vi "construct.vi"(8 "error in (no error)":errorcluster, 9 "configuration name":string, 10 "load config file?":bool=TRUE, 11 "GenericPlugin in":refnum<class "ScanHeadMH100729FPGA.lvclass">) -> (0 "error out":errorcluster, 3 "GenericPlugin out":refnum<class "ScanHeadMH100729FPGA.lvclass">)   [LabVIEW 2010, in "ScanHeadMH100729FPGA.lvclass"]
uses:
  ScanHeadMH100729FPGA.lvclass
  GenericScanHead/GenericScanHead/GenericScanHead.lvclass
  ScanHeadMH100729FPGA.lvclass/ScanHeadMH100729FPGA.ctl
  common/classes/ErrorController/ErrorController/class_data.vi
  common/classes/GenericComponent/GenericComponent/GenericComponent.lvclass
  common/classes/ErrorController/ErrorController/ErrorController.lvclass
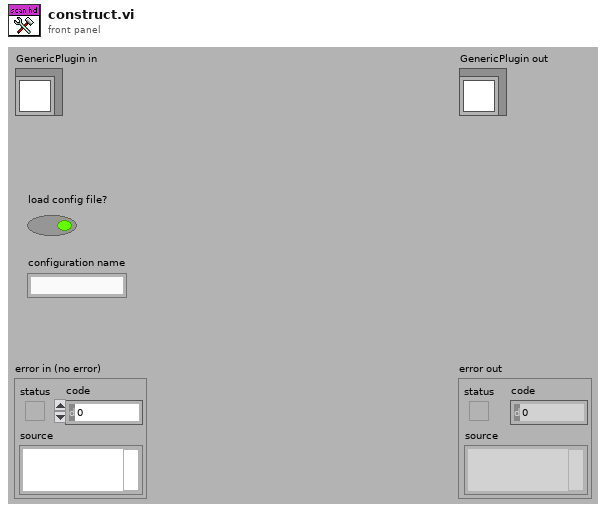
[diagram p1: front panel]
types:
  T1 = typedef "plugin_specification.ctl" = cluster{"class path":string, "configuration":string, "label":string, "settings name":string}
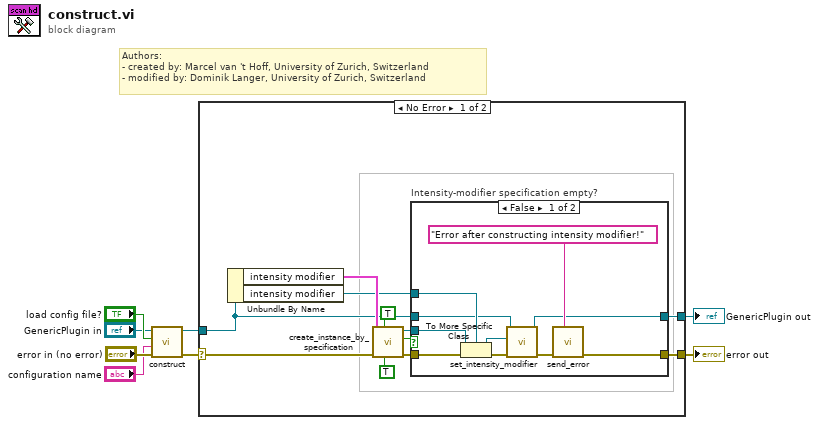
[diagram p0: block diagram]
diagram:
  # "Authors: \n- created by: Marcel van 't Hoff, University of Zurich, Switzerland\n- modified by: Dominik Langer, University of Zurich, Switzerland"
  n1 = call-parent "construct.vi"("error in (no error)"="error in (no error)", "configuration name"="configuration name", "load config file?"="load config file?", "GenericPlugin in"="GenericPlugin in") -> ("error out"=w4:errorcluster, "GenericPlugin out"=w1:refnum<class "ScanHeadMH100729FPGA.lvclass">)  [unwired: 6 in]
  n2 = case shown="No Error" w4 {
    selector: w4 -> [w12 w33]
    tunnel: [w15 w33] -> w3
    tunnel: [w9 w32] -> w2
    tunnel: w1 -> [w10 w32]
    frame No Error {
      n3 = Unbundle By Name(w10) -> ("intensity modifier"=w19:T1, "intensity modifier"=w11:refnum<class "GenericAnalogOut.lvclass">)
      n4 = call "create_instance_by_specification.vi"("be tolerant against empty specification?"=TRUE, "call constructor?"=TRUE, "error in (no error)"=w12, "component specification"=w19) -> ("error out"=w18:errorcluster, "empty specification!"=w13:bool, "GenericPlugin out"=w17:refnum<class "GenericComponent.lvclass">)  [unwired: 5 in]
      n5 = case "Intensity-modifier specification empty?" shown="False" w13 {
        tunnel: w18 -> [w29 w31]
        tunnel: w17 -> [w28 _]
        tunnel: [w23 w31] -> w15
        tunnel: [w22 w30] -> w9
        tunnel: w11 -> [w21 _]
        tunnel: w10 -> [w20 w30]
        frame False {
          n6 = To More Specific Class(target class=w21, reference=w28, error in=w29) -> (specific class reference=w27:refnum<class "GenericAnalogOut.lvclass">, error out=w26:errorcluster)
          n7 = call-dynamic "set_intensity_modifier.vi"("error in (no error)"=w26, "intensity modifier"=w27, "ScanHeadMH100729FPGA in"=w20) -> ("error out"=w25:errorcluster, "ScanHeadMH100729FPGA out"=w22:refnum<class "ScanHeadMH100729FPGA.lvclass">)  [unwired: 7 in]
          n8 = call "send_error.vi"("additional message"="Error after constructing intensity modifier!", "error in (no error)"=w25) -> ("error out"=w23:errorcluster)  [unwired: 9 in]
        }
        frame True {
        }
      }
    }
    frame Error {
    }
  }
  "error out" <- w3
  "GenericPlugin out" <- w2
